vi "OperationCallDVR.vi"(8 "event source":refnum<user-event>, 9 "user event out":refnum<user-event>, 10 "Sub Panel":refnum<vi>, 11 "data value reference in":refnum<data-value>) -> (3 "data value reference out":refnum<data-value>)   [LabVIEW 2023, in "Arithmetic.lvclass"]
doc: "Gets the reference of the selected instance in the tree and loads the corresponding operation UI in the Subpanel."
uses:
  Arithmetic.lvclass
panel:
  out "error out":errorcluster
  in  "error in (no error)":errorcluster
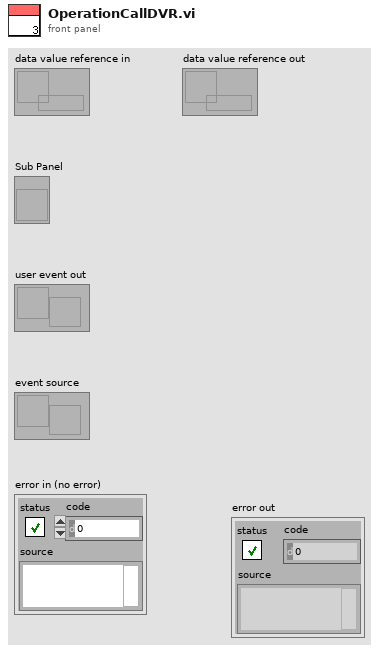
[diagram p1: front panel]
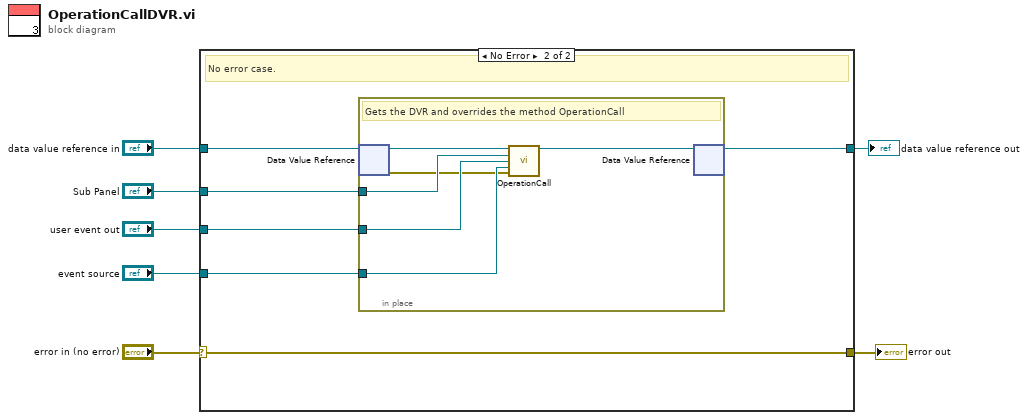
[diagram p0: block diagram]
diagram:
  n1 = case shown="No Error" "error in (no error)" {
    selector: "error in (no error)" -> [w9 w15]
    tunnel: [w9 w15] -> w6
    tunnel: "data value reference in" -> [w8 w14]
    tunnel: [w8 w13] -> w4
    tunnel: "Sub Panel" -> [_ w12]
    tunnel: "user event out" -> [_ w11]
    tunnel: "event source" -> [_ w10]
    frame Error {
      # "Wire the error cluster across even in the \"No Error\"\ncase so that warnings get propagated."
      # "Error Case."
    }
    frame No Error {
      # "No error case."
      n2 = in-place {
        in-place-border: w12 -> [w20]
        in-place-border: w11 -> [w19]
        in-place-border: w10 -> [w18]
        # "Gets the DVR and overrides the method OperationCall"
        n3 = in-place-dvr #1(w14) -> (w21:refnum<class "Arithmetic.lvclass">, w16:errorcluster)
        n4 = call-dynamic "OperationCall.vi"("Arithmetic in"=w21, "Sub Panel"=w20, "user event out"=w19, "event source"=w18, "error in (no error)"=w16) -> ("Arithmetic out"=w17:refnum<class "Arithmetic.lvclass">)  [unwired: 9 in, 1 out]
        n5 = in-place-dvr #1(w17) -> (w13:refnum<data-value>)  [unwired: 1 out]
      }
    }
  }
  "error out" <- w6
  "data value reference out" <- w4
